vi "Decode Multiple (Greyscale).vi"(8 "error in (no error)":errorcluster, 9 "Detections":T1[](array[typedef]), 10 "Greyscale Image in":T3, 11 "QR Code Detector in":refnum<class "QR Code Detector.lvclass">) -> (0 "error out":errorcluster, 2 "Data":string[](array[string]), 3 "QR Code Detector":refnum<class "QR Code Detector.lvclass">)   [LabVIEW 2020, in "feature_detection.lvlib" / "QR Code Detector.lvclass"]
doc: "Decode Multiple QR Codes in an image at the locations specified."
uses:
  QR Code Detector.lvclass
  image/Greyscale Image.ctl
  common/Image Points Quad (Float).ctl
  common/Image Point (Float).ctl
  QR Code Detector.lvclass/QR Code Detector.ctl
  3b41aeaf-0755-48ac-92a1-e7e342c08438.vi
  <vilib>/Utility/error.llb/Error Cluster From Error Code.vi
  common/common.lvlib
  image/image.lvlib
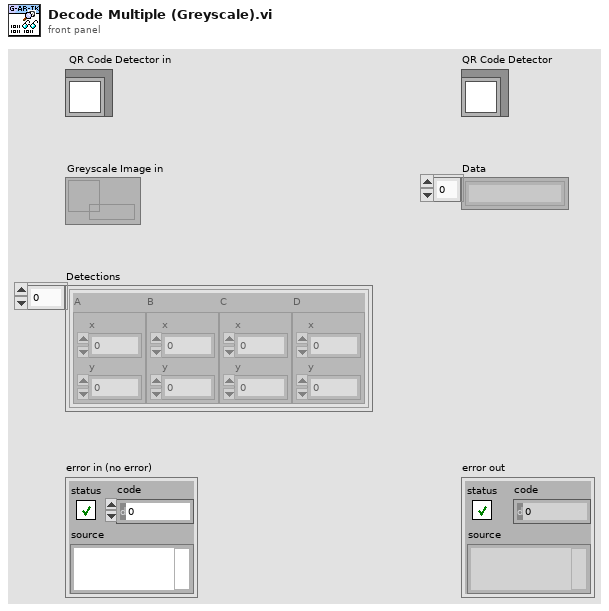
[diagram p1: front panel]
types:
  T1 = typedef "common.lvlib/Image Points Quad (Float).ctl" = cluster{"A":T2, "B":T2, "C":T2, "D":T2}
  T2 = typedef "common.lvlib/Image Point (Float).ctl" = cluster{"x":dbl, "y":dbl}
  T3 = typedef "image.lvlib/Greyscale Image.ctl" = refnum<data-value>
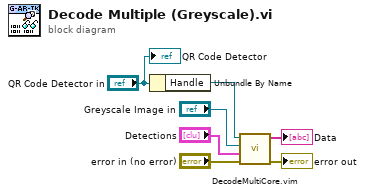
[diagram p0: block diagram]
diagram:
  n1 = Unbundle By Name("QR Code Detector in") -> ("Handle"=w5:refnum<data-value>)
  n2 = call "DecodeMultiCore.vim"("error in (no error)"="error in (no error)", "Detections"="Detections", "Greyscale Image"="Greyscale Image in", "Handle"=w5) -> ("error out"=→"error out":errorcluster, "Info"=→"Data":string[])  [unwired: 6 in]
  "QR Code Detector" <- "QR Code Detector in"
